vi "SemiColonParserFromString(SubVI).vi"(1 "String In":string) -> (0 "String Array Out":string[](array[string]))   [LabVIEW 2018]
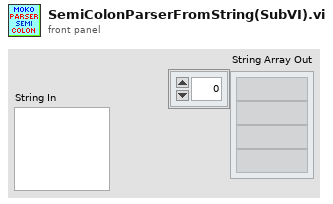
[diagram p1: front panel]
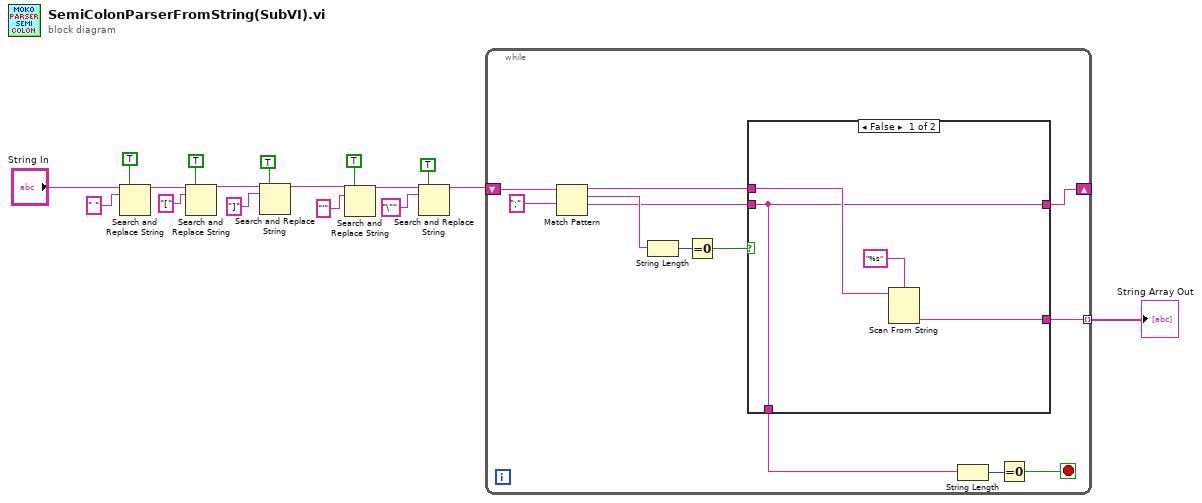
[diagram p0: block diagram]
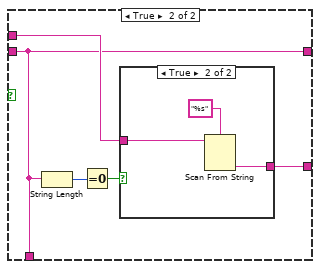
[diagram p2: hidden frame]
diagram:
  n1 = Search and Replace String(replace all?=TRUE ("replace all? (F)"), input string="String In", search string=" ") -> (result string=w14:string)  [unwired: 5 in, 3 out]
  n2 = Search and Replace String(replace all?=TRUE ("replace all? (F)"), input string=w14, search string="[") -> (result string=w12:string)  [unwired: 5 in, 3 out]
  n3 = Search and Replace String(replace all?=TRUE ("replace all? (F)"), input string=w12, search string="]") -> (result string=w2:string)  [unwired: 5 in, 3 out]
  n4 = Search and Replace String(replace all?=TRUE ("replace all? (F)"), input string=w2, search string="'") -> (result string=w6:string)  [unwired: 5 in, 3 out]
  n5 = Search and Replace String(replace all?=TRUE ("replace all? (F)"), input string=w6, search string="\"") -> (result string=w1:string)  [unwired: 5 in, 3 out]
  n6 = while {
    shift-right: [w25] -> _
    shift-left: w1 -> [w29]
    tunnel: [w20] -> w15 mode=indexing
    stop <- w19 stop-if-true
    n7 = Match Pattern(string=w29, regular expression=";" ("string")) -> (before substring=w23:string, match substring=w27:string, after substring=w24:string)  [unwired: 1 in, 1 out]
    n8 = String Length(string=w27) -> (length=w28:i32)
    n9 = Equal To 0?(x=w28) -> (x = 0?=w26:bool)
    n10 = case shown="False" w26 {
      tunnel: [w30 w34] -> w25
      tunnel: w24 -> [w30 w34]
      tunnel: w23 -> [w33 w35]
      tunnel: [w30 w34] -> w22
      tunnel: [w31 w36] -> w20
      frame False {
        n11 = Scan From String(format string="%s", input string=w33) -> (output 1=w31:string)  [unwired: 3 in, 3 out]
      }
      frame True {
        n12 = String Length(string=w34) -> (length=w37:i32)
        n13 = Equal To 0?(x=w37) -> (x = 0?=w38:bool)
        n14 = case shown="True" w38 {
          tunnel: [_ w40] -> w36
          tunnel: w35 -> [_ w39]
          frame False {
          }
          frame True {
            n15 = Scan From String(format string="%s", input string=w39) -> (output 1=w40:string)  [unwired: 3 in, 3 out]
          }
        }
      }
    }
    n16 = String Length(string=w22) -> (length=w21:i32)
    n17 = Equal To 0?(x=w21) -> (x = 0?=w19:bool)
  }
  "String Array Out" <- w15
